vi "test edit.vi"(8 "error in (no error)":errorcluster) -> (0 "error out":errorcluster, 3 "All Passed?":bool)   [LabVIEW 2018, in "labview_json_tests.lvlib"]
uses:
  labview_json_tests.lvlib
panel:
  out "Tests Failed":string[](array[string])
  out "JSON out":string
  out "JSON in":string
  out "Result":variant
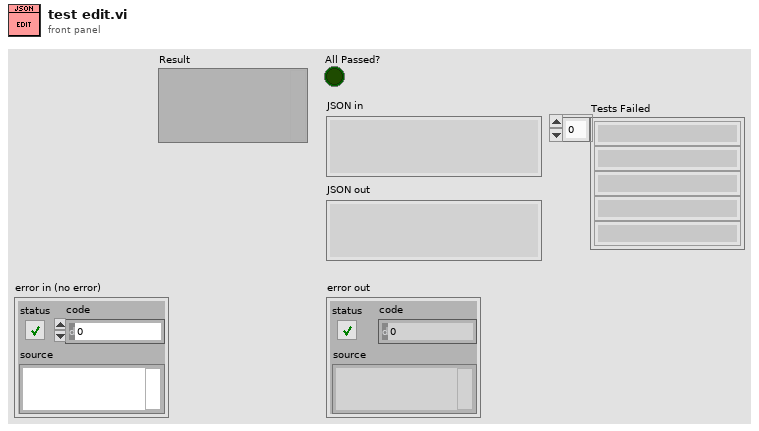
[diagram p1: front panel]
types:
  T1 = enum16{"BooleanFalse", "BooleanTrue", "StringSentence", "StringMultiline", "StringQuoted", "StringEscaped", "IntNumber", "IntMin", "IntMax", "IntI64", "IntI32", "IntI16", "IntI8", "UintNumber", "UintMin", "UintMax", "UintU64", "UintU32", "UintU16", "UintU8", "FloatNumber", "FloatMin", "FloatMax", "FloatZero", "FloatNaN", "FloatExt", "FloatDbl", "FloatSgl", "EnumU32", "EnumU16", "EnumU8", "EnumU32String", "EnumU16String", "EnumU8String", "EnumBadString", "PathAbs", "PathRel", "PathNetwork", "PathFile", "PathEmpty", "PathNaN", "PathCurrentDir", "PathParentDir", "TimeDateTime", "TimeDate", "NullVoid", "NullLVVariant", "NullBoolean", "NullInt", "NullUint", "NullFloat", "NullString", "NullPath", "NullEnum", "NullTime", "NullArray", "NullArrayVoid", "NullArrayLVVariant", "NullObject", "NullObjectVoid", "NullObjectLVVariant", "NullWaveform", "Array1DValues", "Array1DEmpty", "Array1DObject", "Array1DMulti", "Array2DValues", "Array2DEmpty", "Array3DValues", "Array3DEmpty", "ObjectValues", "ObjectEmpty", "ObjectWaveform", "ObjectReorder"}
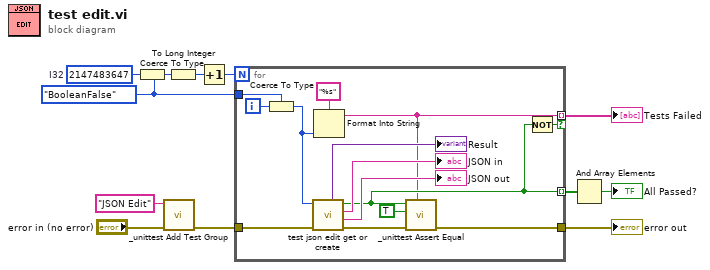
[diagram p0: block diagram]
diagram:
  w2 = T1."BooleanFalse" ("Enum")
  w7 = 2147483647  # I32
  n1 = Coerce To Type(0:w7, 1:w2) -> (2:w8:T1)
  n2 = call "_unittest Add Test Group.vi"("error in (no error)"="error in (no error)", "Test Group"="JSON Edit" ("Test Case")) -> ("error out"=w9:errorcluster)  [unwired: 9 in]
  n3 = To Long Integer(number=w8) -> (32bit integer=w6:i32)
  n4 = Increment(x=w6) -> (x+1=w5:i32)
  n5 = for {
    N: w5 -> [_]
    tunnel: w2 -> [w21]
    tunnel: w9 -> [w26]
    tunnel: [w23] -> w12
    tunnel: [w15] -> w4 mode=indexing
    tunnel: [w13] -> w1 mode=indexing if=w14
    i -> [w25]
    n6 = Coerce To Type(0:w25, 1:w21) -> (2:w16:T1)
    n7 = call "test json edit get or create.vi"("error in (no error)"=w26, "Enum"=w16) -> ("error out"=w24:errorcluster, "JSON out"=→"JSON out":string, "JSON in"=→"JSON in":string, "Passed?"=w15:bool, "Result"=→"Result":variant)  [unwired: 5 in]
    n8 = Format Into String(format string="%s", w16) -> (resulting string=w13:string)  [unwired: 2 in, 1 out]
    n9 = call "_unittest Assert Equal.vi"("Test Name"=w13, "error in (no error)"=w24, "Expected Value"=TRUE, "Actual Value"=w15) -> ("error out"=w23:errorcluster)  [unwired: 5 in, 2 out]
    n10 = Not(x=w15) -> (.not. x?=w14:bool)
  }
  "error out" <- w12
  "Tests Failed" <- w1
  n11 = And Array Elements(Boolean array=w4) -> (logical AND=→"All Passed?":bool)
